vi "Get Attribute - 1D Array Boolean.vi"(8 "error in (no error)":errorcluster, 9 "Default Value (empty)":bool[](array[boolean]), 10 "Key":string, 11 "YAML Parser in":refnum<class "YAML Parser.lvclass">) -> (0 "error out":errorcluster, 1 "Is Null?":bool, 2 "Value":bool[](array[boolean]), 3 "YAML Parser out":refnum<class "YAML Parser.lvclass">)   [LabVIEW 2015, in "YAML Parser.lvclass"]
uses:
  YAML Parser.lvclass
  <vilib>/Utility/error.llb/Error Cluster From Error Code.vi
  <vilib>/ErrorRing/Error Ring.xnode
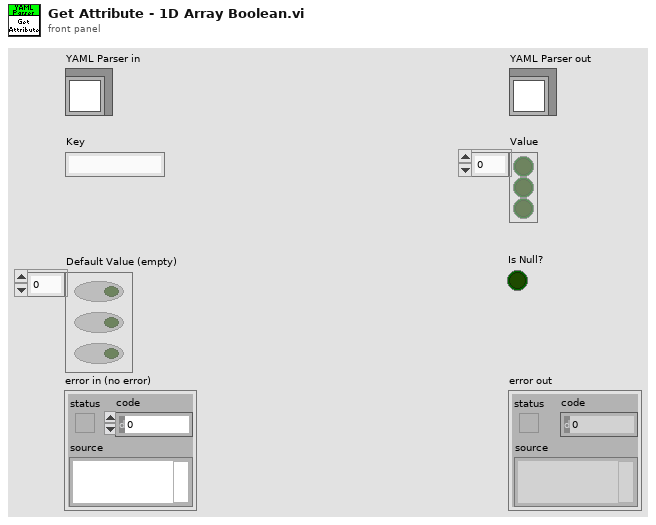
[diagram p1: front panel]
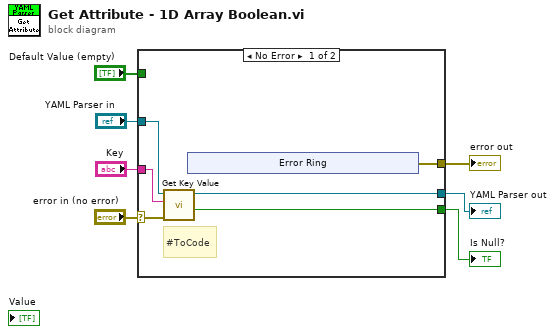
[diagram p0: block diagram]
diagram:
  n1 = case shown="No Error" "error in (no error)" {
    selector: "error in (no error)" -> [w13 w20]
    tunnel: [w8 w20] -> w6
    tunnel: [w11 w19] -> w4
    tunnel: "YAML Parser in" -> [w12 w19]
    tunnel: "Default Value (empty)" -> [_ _]
    tunnel: "Key" -> [w10 _]
    tunnel: [w9 _] -> w1
    frame No Error {
      # "#ToCode"
      n2 = call "Get Key Value.vi"("error in (no error)"=w13, "Key"=w10, "YAML Parser in"=w12) -> ("Is Null?"=w9:bool, "YAML Parser out"=w11:refnum<class "YAML Parser.lvclass">)  [unwired: 5 in, 2 out]
      n3 = xnode "Error Ring"() -> ("error out"=w8:errorcluster)
    }
    frame Error {
    }
  }
  "error out" <- w6
  "YAML Parser out" <- w4
  "Is Null?" <- w1
